vi "Initialize_DMM.vi"(8 "error in (no error)":errorcluster, 10 "DMM_Initialize":T1, 11 "niDMM in":refnum<class "niDMM.lvclass">) -> (0 "error out":errorcluster, 3 "niDMM out":refnum<class "niDMM.lvclass">)   [LabVIEW 2020, in "niDMM.lvclass"]
uses:
  niDMM.lvclass
  DMM_Base/Typedef/DMM_Initialize.ctl
  <vilib>/MeasurementLink/MeasurementLink Session Management V1/Session Reservation/Initialize and Close Session Behavior.ctl
  niDMM.lvclass/niDMM.ctl
  <vilib>/MeasurementLink/MeasurementLink niDMM/Initialize Sessions - 1Sess.vi
  <vilib>/MeasurementLink/MeasurementLink niDMM/MeasurementLink niDMM.lvlib
  <vilib>/MeasurementLink/MeasurementLink Session Management V1/Session Reservation/Session Reservation.lvclass
  DMM_Base/DMM_Base.lvclass
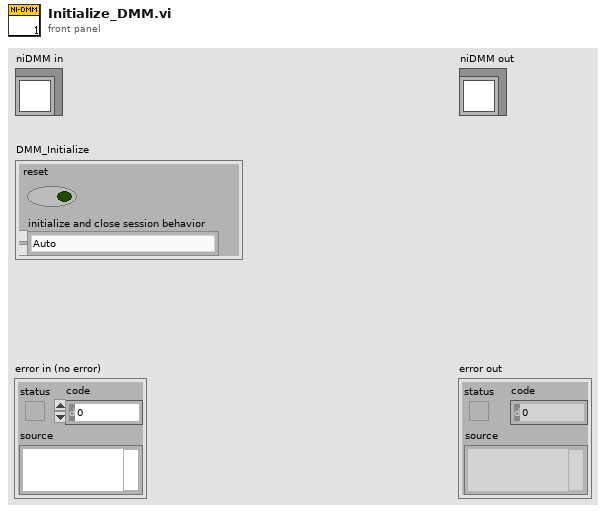
[diagram p1: front panel]
types:
  T1 = typedef "DMM_Base.lvclass/DMM_Initialize.ctl" = cluster{"initialize and close session behavior":T2, "reset":bool}
  T2 = typedef "MeasurementLink Session Management V1.lvlib/Session Reservation.lvclass/Initialize and Close Session Behavior.ctl" = enum16{"Auto", "Initialize and Close", "Attach and Detach", "Initialize and Detach", "Attach and Close"}
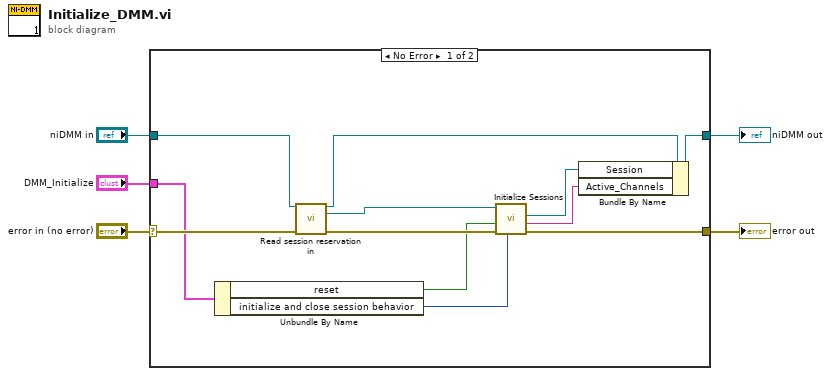
[diagram p0: block diagram]
diagram:
  n1 = case shown="No Error" "error in (no error)" {
    selector: "error in (no error)" -> [w15 w19]
    tunnel: "niDMM in" -> [w14 w18]
    tunnel: "DMM_Initialize" -> [w13 _]
    tunnel: [w10 w19] -> w2
    tunnel: [w8 w18] -> w1
    frame No Error {
      n2 = Unbundle By Name(w13) -> ("reset"=w11:bool, "initialize and close session behavior"=w12:T2)
      n3 = call-dynamic "Read session reservation in.vi"("AbstractDMM in"=w14, "error in (no error)"=w15) -> ("AbstractDMM out"=w9:refnum<class "niDMM.lvclass">, "MeasurementLink Session Management V1.lvlib:Session Reservation.lvclass"=w17:refnum<class "Session Reservation.lvclass">, "error out"=w16:errorcluster)  [unwired: 11 in]
      n4 = call-poly <vilib>:"Initialize Sessions.vi"("initialize and close session behavior"=w12, "error in"=w16, "reset"=w11, "session reservation in"=w17) -> ("error out"=w10:errorcluster, "channel list"=w6:string, "session"=w7:refnum<k15>)  [unwired: 4 in, 1 out]
      n5 = Bundle By Name(cluster=w9, "Session"=w7, "Active_Channels"=w6) -> (w8:refnum<class "niDMM.lvclass">)
    }
    frame Error {
    }
  }
  "error out" <- w2
  "niDMM out" <- w1
